vi "network测试版.vi"() -> ()   [LabVIEW 2011]
uses:
  R&S/RS.lvclass
  keysight/keysight.lvclass
  ctl/state.ctl
  network/network.lvclass
  Globle/Global.vi
panel:
  in  "测试":bool
  in  "单通道测试":bool
  in  "Limit":dbl
  in  "connect":bool
  in  "Remote Address":refnum<visa-resource-name>="TCPIP0::192.168.1.253::inst0::INSTR"
  in  "Points":i32=401 caption="测量点数"
  in  "IF_Band":dbl=10.0 format="%.3f"
  in  "Stop":dbl=3900.0 format="%.3f"
  in  "Start":dbl=600.0 format="%.3f"
  in  "网分tab":enum32{"Keysight", "R&S"}(tab)
  in  "out":i32=4
  in  "in":i32=128
  out "消息":string
  in  "stop":bool
  # "MHz"
  # "MHz"
  # "Point"
  # "kHz"
  # "dB"
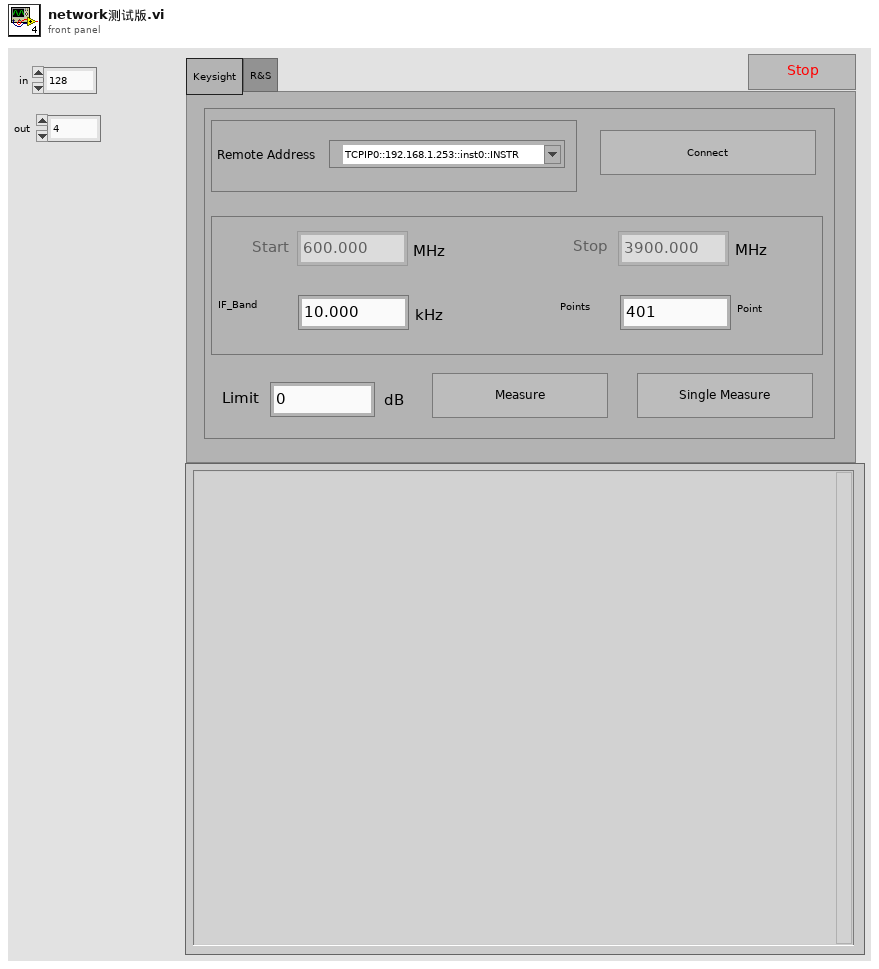
[diagram p1: front panel]
types:
  T1 = typedef "state.ctl" = enum16{"Idle", "直通基准测试", "校准基准测试", "校准直接测试", "导出基准数据", "导出差值数据"}
  T2 = typedef "Database.lvclass/database_Method.ctl" = enum16{"初始化", "查询", "关闭"}
  T3 = typedef "数据源.ctl" = string
  T4 = enum16{"Left Button", "Center Button", "Right Button", "Window Close"}
  T5 = typedef "FIFOs STM Multi-client Example.ctl" = cluster{"命令":refnum<queue>, "时钟命令反馈":refnum<queue>, "广播":refnum<queue>, "命令反馈":refnum<queue>, "时钟命令":refnum<queue>, "TIME-1":refnum<queue>, "TIME-2":refnum<queue>, "TIME-3":refnum<queue>, "TIME-4":refnum<queue>, "命令 2":refnum<queue>, "OUT切换":refnum<queue>, "命令反馈 2":refnum<queue>}
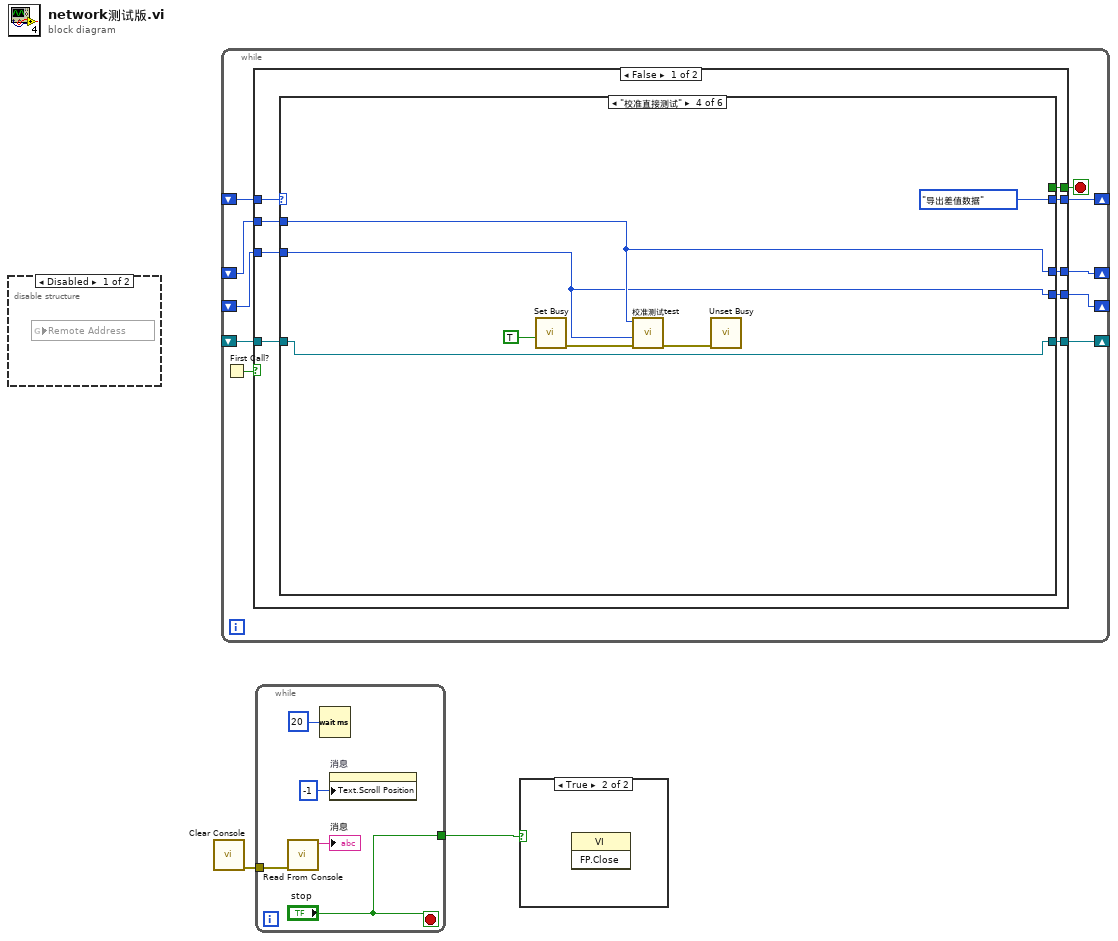
[diagram p0: block diagram]
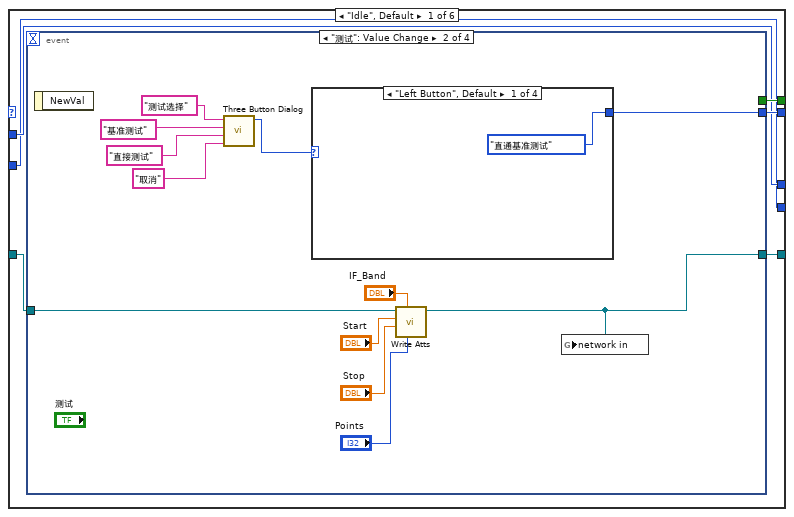
[diagram p4: hidden frame]
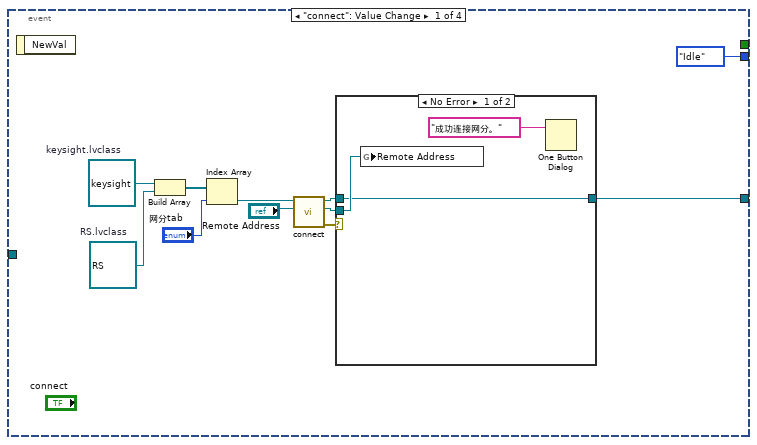
[diagram p5: hidden frame]
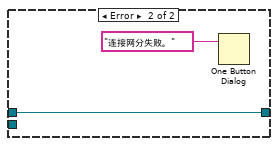
[diagram p6: hidden frame]
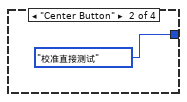
[diagram p7: hidden frame]
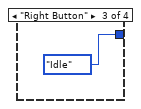
[diagram p8: hidden frame]
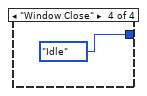
[diagram p9: hidden frame]
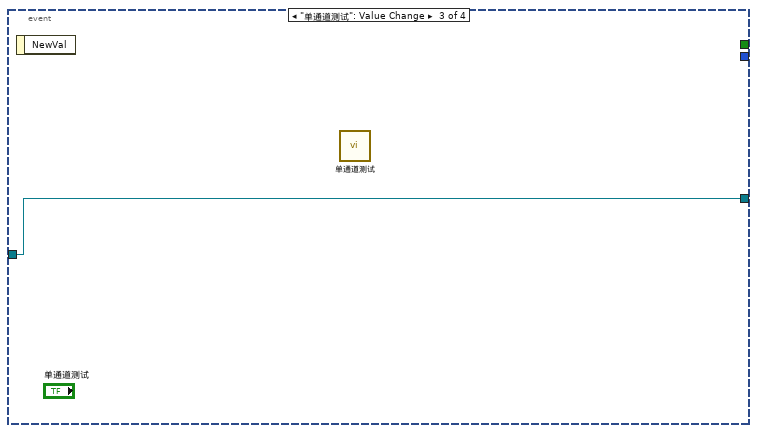
[diagram p10: hidden frame]
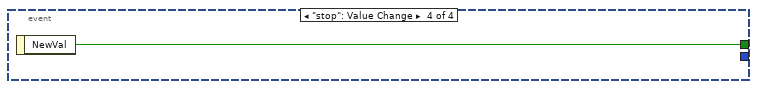
[diagram p11: hidden frame]
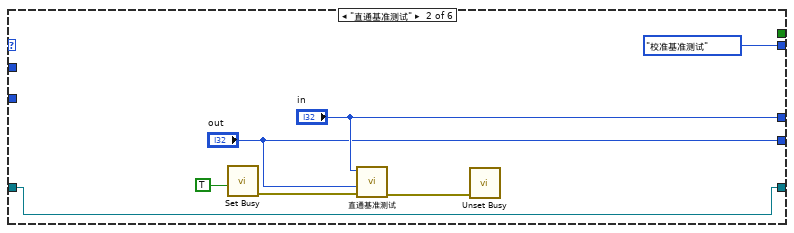
[diagram p12: hidden frame]
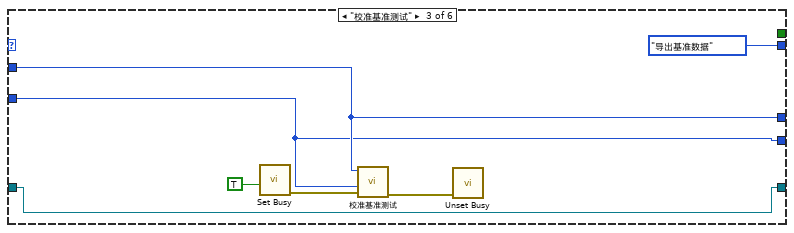
[diagram p13: hidden frame]
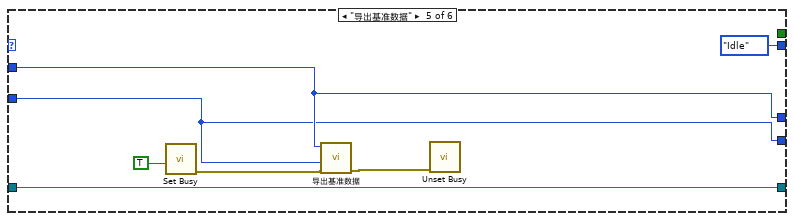
[diagram p14: hidden frame]
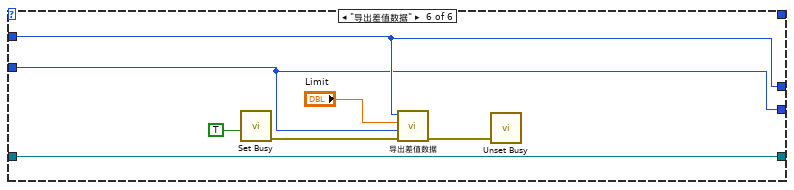
[diagram p15: hidden frame]
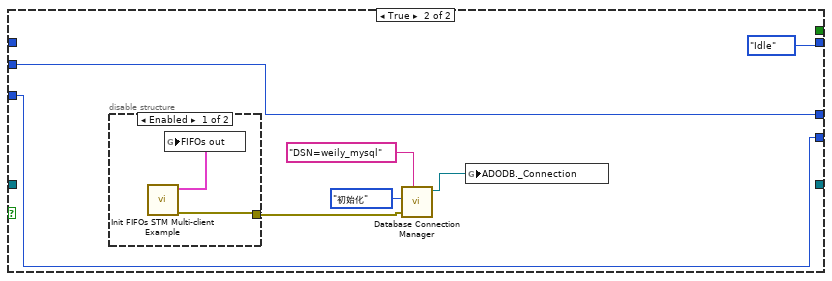
[diagram p16: hidden frame]
diagram:
  n1 = disable-structure shown="Disabled" {
    frame Disabled {
      n2 = global read "Global.vi" "Remote Address"() -> ()  [unwired: 1 in]
    }
    frame Enabled {
    }
  }
  n3 = call "Clear Console.vi"() -> ("error out"=w2:errorcluster)  [unwired: 11 in]
  n4 = while {
    shift-right: [w10] -> _
    shift-left: _ -> [w11]
    shift-right: [w9] -> _
    shift-left: _ -> [w7]
    shift-right: [w6] -> _
    shift-left: _ -> [w4]
    shift-right: [w5] -> _
    shift-left: _ -> [w3]
    stop <- w12 stop-if-true
    n5 = First Call?() -> (First Call?: T/F=w8:bool)
    n6 = case shown="False" w8 {
      tunnel: [w21 _] -> w12
      tunnel: w11 -> [w20 _]
      tunnel: [w19 state."Idle" ("Enum")] -> w10
      tunnel: [w18 _] -> w9
      tunnel: w7 -> [w17 _]
      tunnel: w4 -> [w16 w98]
      tunnel: w3 -> [w15 w97]
      tunnel: [w14 w98] -> w6
      tunnel: [w13 w97] -> w5
      frame False {
        n7 = case shown="\"校准直接测试\"" w20 {
          tunnel: [w27 _ _ _ _ _] -> w21
          tunnel: [w26 state."校准基准测试" ("Enum") state."导出基准数据" ("Enum") state."导出差值数据" ("Enum") state."Idle" ("Enum") _] -> w19
          tunnel: [w25 w64 w71 w78 w85 w92] -> w18
          tunnel: w17 -> [w24 w64 w71 w78 w85 w92]
          tunnel: w16 -> [w23 _ w70 w77 w84 w91]
          tunnel: w15 -> [w22 _ w69 w76 w83 w90]
          tunnel: [w23 "in" w70 w77 w84 w91] -> w14
          tunnel: [w22 "out" w69 w76 w83 w90] -> w13
          frame "Idle", Default {
            n8 = event shown="[1] \"测试\": Value Change" {
              selector: _ -> [_ _ _ _]
              dyn-events: _ -> [_ _ _ _]
              timeout: _ -> [_ _ _ _]
              tunnel: [_ _ _ w61] -> w27
              tunnel: [state."Idle" ("Enum") w50 _ _] -> w26
              tunnel: [w28 w44 w60 _] -> w25
              tunnel: w24 -> [_ w45 w60 _]
              event "connect": Value Change {
                w32 = refnum<class "RS.lvclass"> refnum  # RS.lvclass
                w31 = refnum<class "keysight.lvclass"> refnum  # keysight.lvclass
                n9 = event-data() -> ()  [unwired: 1 in, 1 out]
                n10 = Build Array(w31, w32) -> (w30:refnum<class "network.lvclass">[])
                n11 = Index Array(array=w30, index="网分tab") -> (element=w37:refnum<class "network.lvclass">)
                n12 = call-dynamic "connect.vi"("VISA resource name"="Remote Address", "network in"=w37) -> ("error out"=w36:errorcluster, "VISA resource name out"=w33:refnum<visa-resource-name>, "network out"=w29:refnum<class "network.lvclass">)  [unwired: 7 in]
                n13 = case shown="No Error" w36 {
                  tunnel: w33 -> [w40 _]
                  tunnel: w29 -> [w39 w42]
                  tunnel: [w39 w42] -> w28
                  frame No Error {
                    n14 = global write "Global.vi" "Remote Address"(w40) -> ()
                    n15 = One Button Dialog(message="成功连接网分。") -> ()  [unwired: 1 in, 1 out]
                  }
                  frame Error {
                    n16 = One Button Dialog(message="连接网分失败。") -> ()  [unwired: 1 in, 1 out]
                  }
                }
              }
              event "测试": Value Change {
                n17 = event-data() -> ()  [unwired: 1 in, 1 out]
                n18 = call <vilib>:"Three Button Dialog.vi"("Right Button Text (\"Cancel\")"="取消" ("Right Button Text (\"Cancel\")"), "Center Button Text (\"No\")"="直接测试" ("message"), "Left Button Text (\"Yes\")"="基准测试" ("message"), "message"="测试选择") -> ("Which Button?"=w51:T4)  [unwired: 7 in]
                n19 = case shown="\"Left Button\", Default" w51 {
                  tunnel: [state."直通基准测试" ("Enum") state."校准直接测试" ("Enum") state."Idle" ("Enum") state."Idle" ("Enum")] -> w50
                  frame "Left Button", Default {
                  }
                  frame "Center Button" {
                  }
                  frame "Right Button" {
                  }
                  frame "Window Close" {
                  }
                }
                n20 = call-dynamic "Write Atts.vi"("Points"="Points", "IF_Band"="IF_Band", "Stop"="Stop", "Start"="Start", "network in"=w45) -> ("network out"=w44:refnum<class "network.lvclass">)  [unwired: 5 in, 1 out]
                n21 = global write "Global.vi" "network in"(w44) -> ()
              }
              event "单通道测试": Value Change {
                n22 = event-data() -> ()  [unwired: 1 in, 1 out]
                n23 = call "单通道测试.vi"() -> ()  [unwired: 20 in]
              }
              event "stop": Value Change {
                n24 = event-data() -> ("NewVal"=w61:bool)  [unwired: 1 in]
              }
            }
          }
          frame "直通基准测试" {
            n25 = call <vilib>:"Set Busy.vi"("disable click? (T)"=TRUE) -> ("error out"=w66:errorcluster)  [unwired: 9 in, 1 out]
            n26 = call "直通基准测试.vi"("error in (no error)"=w66, "out"="out", "in"="in") -> ("error out"=w65:errorcluster)  [unwired: 8 in]
            n27 = call <vilib>:"Unset Busy.vi"("error in (no error)"=w65) -> ()  [unwired: 10 in, 1 out]
          }
          frame "校准基准测试" {
            n28 = call <vilib>:"Set Busy.vi"("disable click? (T)"=TRUE) -> ("error out"=w74:errorcluster)  [unwired: 9 in, 1 out]
            n29 = call "校准基准测试.vi"("error in (no error)"=w74, "out"=w69, "in"=w70) -> ("error out"=w73:errorcluster)  [unwired: 8 in]
            n30 = call <vilib>:"Unset Busy.vi"("error in (no error)"=w73) -> ()  [unwired: 10 in, 1 out]
          }
          frame "校准直接测试" {
            n31 = call <vilib>:"Set Busy.vi"("disable click? (T)"=TRUE) -> ("error out"=w80:errorcluster)  [unwired: 9 in, 1 out]
            n32 = call "校准测试test.vi"("error in (no error)"=w80, "out"=w76, "in"=w77) -> ("error out"=w79:errorcluster)  [unwired: 8 in]
            n33 = call <vilib>:"Unset Busy.vi"("error in (no error)"=w79) -> ()  [unwired: 10 in, 1 out]
          }
          frame "导出基准数据" {
            n34 = call <vilib>:"Set Busy.vi"("disable click? (T)"=TRUE) -> ("error out"=w87:errorcluster)  [unwired: 9 in, 1 out]
            n35 = call "导出基准数据.vi"("error in"=w87, "OUT"=w83, "IN"=w84) -> ("error out"=w86:errorcluster)  [unwired: 8 in]
            n36 = call <vilib>:"Unset Busy.vi"("error in (no error)"=w86) -> ()  [unwired: 10 in, 1 out]
          }
          frame "导出差值数据" {
            n37 = call <vilib>:"Set Busy.vi"("disable click? (T)"=TRUE) -> ("error out"=w94:errorcluster)  [unwired: 9 in, 1 out]
            n38 = call "导出差值数据.vi"("error in"=w94, "COM"=w90, "阀值"="Limit", "IN"=w91) -> ("error out"=w95:errorcluster)  [unwired: 7 in]
            n39 = call <vilib>:"Unset Busy.vi"("error in (no error)"=w95) -> ()  [unwired: 10 in, 1 out]
          }
        }
      }
      frame True {
        n40 = disable-structure shown="Enabled" {
          disable-tunnel: [w104 _] -> w100
          frame Enabled {
            n41 = call "Init FIFOs STM Multi-client Example.vi"() -> ("error out"=w104:errorcluster, "FIFOs out"=w105:T5)  [unwired: 10 in]
            n42 = global write "Global.vi" "FIFOs out"(w105) -> ()
          }
          frame Disabled {
          }
        }
        n43 = call "Database Connection Manager.vi"("ConnectionString"=T3 "DSN=weily_mysql" ("数据源"), "error in (no error)"=w100, "Method"=database_Method."初始化") -> ("ADODB._Connection Out"=w99:refnum<k7>)  [unwired: 5 in, 3 out]
        n44 = global write "Global.vi" "ADODB._Connection"(w99) -> ()
      }
    }
  }
  n45 = while {
    tunnel: w2 -> [w109]
    tunnel: ["stop"] -> w1
    stop <- "stop" stop-if-true
    n46 = call "Read From Console.vi"("error in (no error)"=w109) -> ("Output"=→"消息":string)  [unwired: 9 in, 1 out]
    n47 = Wait (ms)(milliseconds to wait=u32 20) -> ()  [unwired: 1 out]
    n48 = property on="消息" class="Str"("Text.Scroll Position"=i8 -1 ("milliseconds to wait")) -> ()  [unwired: 2 in, 2 out]
  }
  n49 = case shown="True" w1 {
    frame False {
    }
    frame True {
      n50 = invoke class="VI" method="FP.Close"() -> ()  [unwired: 3 in, 3 out]
    }
  }
